vi "Test Assert Event to JSON.vi"(9 "indent level":i32, 10 "Test Event":T1={"Name"="", "Passed"=FALSE, "Call Chain"=[], "Test Error"={"status"=FALSE, "code"=0, "source"=""}, "Time Stamp"=timestamp(0 s since 1904-01-01), "Unique Assert ID"="", "Test ID"="", "Execution time (s)"=-1.0, "Verbose Explanation"=""}) -> (2 "<JSON>Assertion Event":string)   [LabVIEW 2013, in "Caraya.lvlib" / "Test Result.lvclass"]
uses:
  Test Result.lvclass
  Assert Event Data.ctl
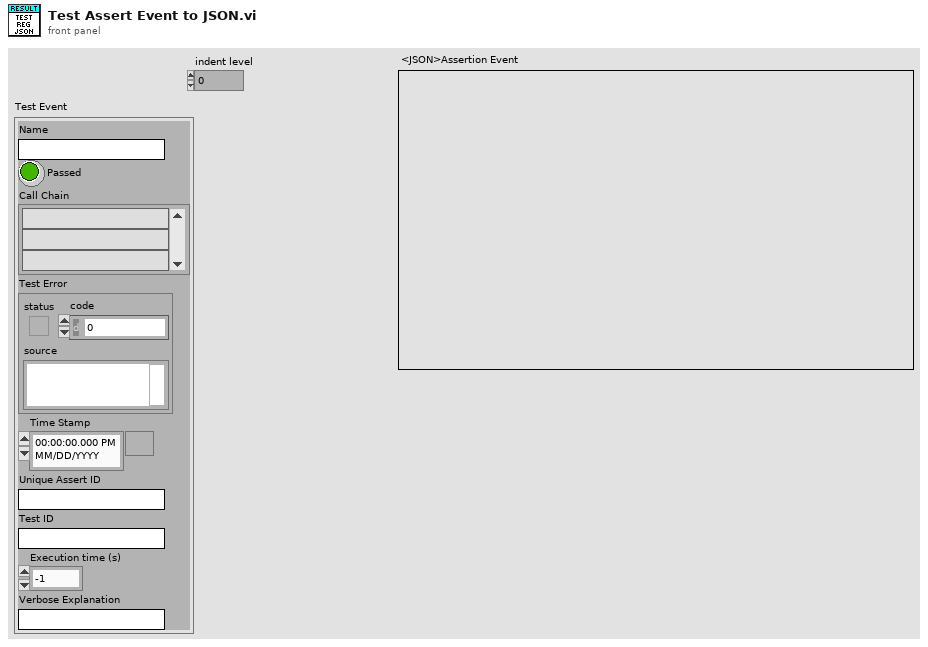
[diagram p1: front panel]
types:
  T1 = typedef "Caraya.lvlib/Test Result.lvclass/Assert Event Data.ctl" = cluster{"Name":string, "Passed":bool, "Call Chain":string[], "Test Error":errorcluster, "Time Stamp":timestamp, "Unique Assert ID":string, "Test ID":string, "Execution time (s)":dbl, "Verbose Explanation":string}
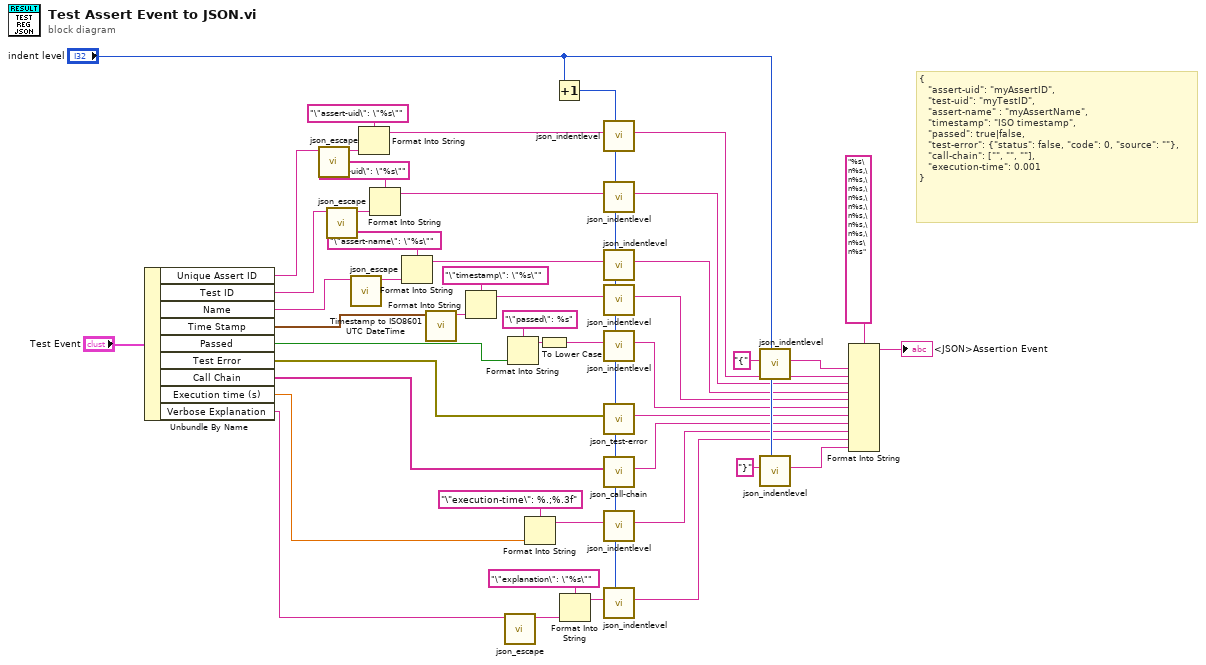
[diagram p0: block diagram]
diagram:
  # "{\n   \"assert-uid\": \"myAssertID\",\n   \"test-uid\": \"myTestID\",\n   \"assert-name\" : \"myAssertName\",\n   \"timestamp\": \"ISO timestamp\",\n   \"passed\": true|false,\n   \"test-error\": {\"status\": false, \"code\": 0, \"source\": \"\"},\n   \"call-chain\": [\"\", \"\", \"\"],\n   \"execution-time\": 0.001\n}"
  n1 = Unbundle By Name("Test Event") -> ("Unique Assert ID"=w31:string, "Test ID"=w27:string, "Name"=w23:string, "Time Stamp"=w44:timestamp, "Passed"=w17:bool, "Test Error"=w4:errorcluster, "Call Chain"=w5:string[], "Execution time (s)"=w7:dbl, "Verbose Explanation"=w11:string)
  n2 = call "json_escape.vi"("string"=w31) -> ("escaped string"=w30:string)  [unwired: 10 in]
  n3 = call "json_escape.vi"("string"=w27) -> ("escaped string"=w29:string)  [unwired: 10 in]
  n4 = call "json_escape.vi"("string"=w23) -> ("escaped string"=w24:string)  [unwired: 10 in]
  n5 = Format Into String(format string="\"assert-uid\": \"%s\"", w30) -> (resulting string=w32:string)  [unwired: 2 in, 1 out]
  n6 = Format Into String(format string="\"test-uid\": \"%s\"", w29) -> (resulting string=w26:string)  [unwired: 2 in, 1 out]
  n7 = Format Into String(format string="\"assert-name\": \"%s\"", w24) -> (resulting string=w22:string)  [unwired: 2 in, 1 out]
  n8 = call <vilib>:"Timestamp to ISO8601 UTC DateTime.vi"("Timestamp (now)"=w44) -> ("ISO8601 UTC DateTime"=w21:string)  [unwired: 10 in]
  n9 = Format Into String(format string="\"timestamp\": \"%s\"", w21) -> (resulting string=w20:string)  [unwired: 2 in, 1 out]
  n10 = call "json_escape.vi"("string"=w11) -> ("escaped string"=w14:string)  [unwired: 10 in]
  n11 = Format Into String(format string="\"passed\": %s", w17) -> (resulting string=w18:string)  [unwired: 2 in, 1 out]
  n12 = Format Into String(format string="\"execution-time\": %.;%.3f", w7) -> (resulting string=w8:string)  [unwired: 2 in, 1 out]
  n13 = To Lower Case(string=w18) -> (all lower case string=w16:string)
  n14 = Increment(x="indent level") -> (x+1=w2:i32)
  n15 = Format Into String(format string="\"explanation\": \"%s\"", w14) -> (resulting string=w12:string)  [unwired: 2 in, 1 out]
  n16 = call "json_indentlevel.vi"("indent level"=w2, "string"=w32) -> ("indented string"=w38:string)  [unwired: 9 in]
  n17 = call "json_indentlevel.vi"("indent level"=w2, "string"=w26) -> ("indented string"=w37:string)  [unwired: 9 in]
  n18 = call "json_indentlevel.vi"("indent level"=w2, "string"=w22) -> ("indented string"=w36:string)  [unwired: 9 in]
  n19 = call "json_indentlevel.vi"("indent level"=w2, "string"=w20) -> ("indented string"=w35:string)  [unwired: 9 in]
  n20 = call "json_indentlevel.vi"("indent level"=w2, "string"=w16) -> ("indented string"=w34:string)  [unwired: 9 in]
  n21 = call "json_test-error.vi"("indent level"=w2, "error"=w4) -> ("indented string"=w1:string)  [unwired: 9 in]
  n22 = call "json_call-chain.vi"("indent level"=w2, "Call Chain"=w5) -> ("indented string"=w3:string)  [unwired: 9 in]
  n23 = call "json_indentlevel.vi"("indent level"=w2, "string"=w8) -> ("indented string"=w6:string)  [unwired: 9 in]
  n24 = call "json_indentlevel.vi"("indent level"=w2, "string"=w12) -> ("indented string"=w10:string)  [unwired: 9 in]
  n25 = call "json_indentlevel.vi"("indent level"="indent level", "string"="{") -> ("indented string"=w42:string)  [unwired: 9 in]
  n26 = call "json_indentlevel.vi"("indent level"="indent level", "string"="}") -> ("indented string"=w40:string)  [unwired: 9 in]
  n27 = Format Into String(format string="%s\n%s,\n%s,\n%s,\n%s,\n%s,\n%s,\n%s,\n%s,\n%s\n%s", w42, w38, w37, w36, w35, w34, w1, w3, w6, w10, w40) -> (resulting string=→"<JSON>Assertion Event":string)  [unwired: 2 in, 1 out]
